vi "FTW-JSON-Object-DeleteAllElements.vi"(0 "JSON Object":refnum<data-value>, 11 "error in":errorcluster) -> (4 "JSON Object out":refnum<data-value>, 15 "error out":errorcluster)   [LabVIEW 2015]
uses:
  core/FTW-JSON-Core-Structure.ctl
panel:
  # "Inputs"
  # "Outputs"
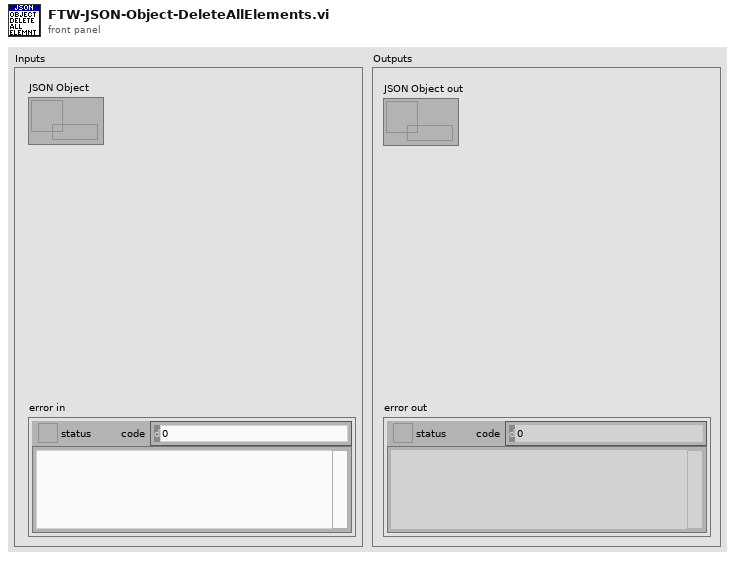
[diagram p1: front panel]
types:
  T1 = typedef "FTW-JSON-Core-Structure.ctl" = cluster{"JSON Object":i64, "Encoding Flags":i64, "Decoding Flags":i64}
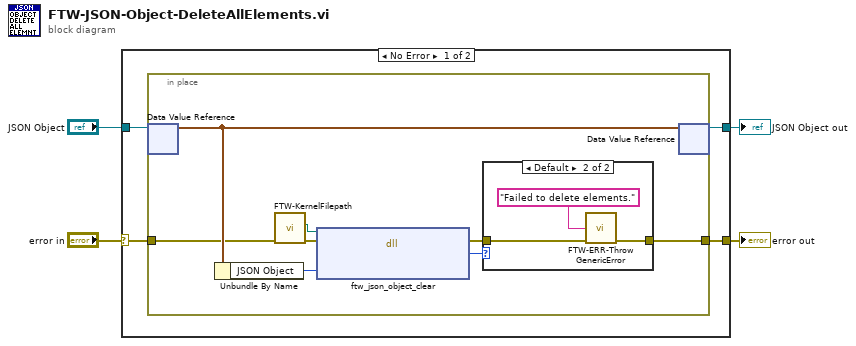
[diagram p0: block diagram]
diagram:
  n1 = case shown="No Error" "error in" {
    selector: "error in" -> [w8 w22]
    tunnel: [w7 w22] -> w4
    tunnel: [w5 w21] -> w2
    tunnel: "JSON Object" -> [w6 w21]
    frame No Error {
      n2 = in-place {
        in-place-border: w8 -> [w11]
        in-place-border: [w12] -> w7
        n3 = in-place-dvr #1(w6) -> (w16:T1)  [unwired: 1 out]
        n4 = Unbundle By Name(w16) -> ("JSON Object"=w15:i64)
        n5 = call "FTW-KernelFilepath.vi"("error in"=w11) -> ("error out"=w10:errorcluster, "Library Filepath"=w9:path)  [unwired: 8 in, 1 out]
        n6 = dll-call lib="?" fn="ftw_json_object_clear"(path in=w9, error in=w10, "JSON Object Pointer"=w15) -> (error out=w13:errorcluster, "Return Value"=w14:i64)  [unwired: 2 in, 1 out]
        n7 = case shown="Default" w14 {
          tunnel: w13 -> [w17 w20]
          tunnel: [w17 w19] -> w12
          frame 0 {
          }
          frame Default {
            n8 = call "FTW-ERR-ThrowGenericError.vi"("Error Message"="Failed to delete elements.", "error in"=w20) -> ("error out"=w19:errorcluster)  [unwired: 13 in]
          }
        }
        n9 = in-place-dvr #1(w16) -> (w5:refnum<data-value>)  [unwired: 1 out]
      }
    }
    frame Error {
    }
  }
  "error out" <- w4
  "JSON Object out" <- w2
